vi "ICM aU64.vi"(9 "Reverse Bytes":bool, 10 "Swap Bytes":bool, 11 "String In":string) -> (1 "Value U64":u64, 2 "Value":dbl, 3 "String Out":string)   [LabVIEW 2018]
doc: "ICM aU64.vi\n\n This VI is used to parse binary data that contains a U64 integer.\n\nThis VI was original part of the OSDS system.\n\nInstrument Communication Module Version 1.0\nSeptember, 2017 Original Code Consulting David Thomson\n www.originalcode.com"
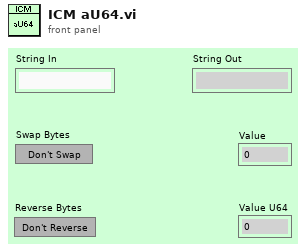
[diagram p1: front panel]
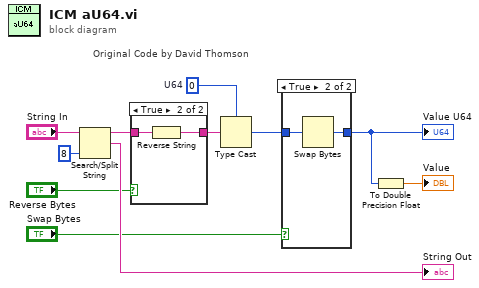
[diagram p0: block diagram]
diagram:
  w9 = u64 0  # U64
  n1 = Search/Split String(string="String In", offset (0)=8) -> (substring before match=w6:string, match + rest of string=→"String Out":string)  [unwired: 2 out]
  n2 = case "Original Code by David Thomson" shown="True" "Reverse Bytes" {
    tunnel: w6 -> [w12 w14]
    tunnel: [w12 w13] -> w5
    frame False {
    }
    frame True {
      n3 = Reverse String(1:w14) -> (0:w13:string)
    }
  }
  n4 = Type Cast(type=w9, x=w5) -> (*(type *) &x=w3:u64)
  n5 = case shown="True" "Swap Bytes" {
    tunnel: w3 -> [w15 w17]
    tunnel: [w15 w16] -> w2
    frame False {
    }
    frame True {
      n6 = Swap Bytes(anything=w17) -> (byte swapped=w16:u64)
    }
  }
  "Value U64" <- w2
  n7 = To Double Precision Float(number=w2) -> (double precision float=→"Value":dbl)
